vi "Set Target Node.vi"(0 "FSM.Graph In":refnum<class "FSM.Graph.lvclass">, 7 "Index":i32) -> (4 "FSM.Graph Out":refnum<class "FSM.Graph.lvclass">)   [LabVIEW 2020, in "FSM.Graph.lvclass"]
uses:
  FSM.Graph.lvclass
  FSM.Graph.lvclass/FSM.Graph.ctl
  FSM.Node/FSM.Node.lvclass/FSM.Node.ctl
  FSM.Node/Write BannerColor.vi
  FSM.Node/Read Shape.vi
  FSM.Node/FSM.Node.lvclass
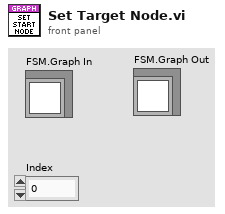
[diagram p1: front panel]
types:
  T1 = typedef "FSM.Node.lvclass/Shape.ctl" = enum16{"Default", "Start", "Action", "End"}
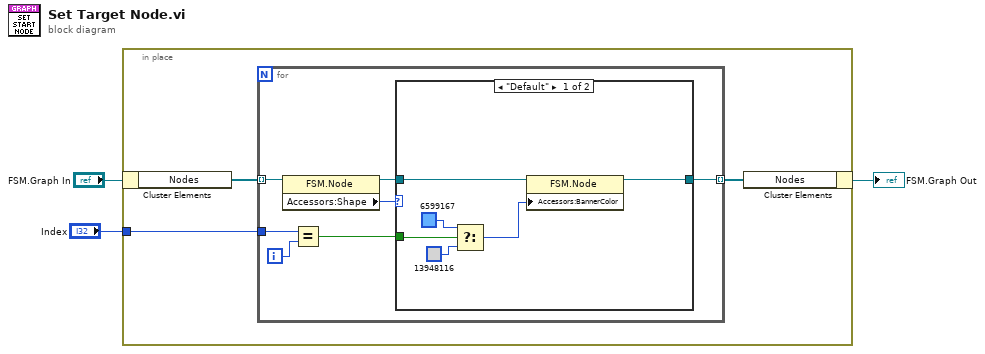
[diagram p0: block diagram]
diagram:
  n1 = in-place {
    in-place-border: "Index" -> [w5]
    n2 = in-place-cluster #1("FSM.Graph In") -> ("Nodes"=w6:refnum<class "FSM.Node.lvclass">[])
    n3 = for {
      tunnel: w6 -> [w12] mode=indexing
      tunnel: w5 -> [w13]
      tunnel: [w7] -> w4 mode=indexing
      i -> [w8]
      n4 = property class="FSM.Node"(reference=w12) -> (reference out=w10:refnum<class "FSM.Node.lvclass">, "Accessors:Shape"=w9:T1)  [unwired: 1 in, 1 out]
      n5 = Equal?(x=w13, y=w8) -> (x = y?=w11:bool)
      n6 = case shown="\"Default\"" w9 {
        tunnel: w10 -> [w19 w20]
        tunnel: [w18 w20] -> w7
        tunnel: w11 -> [w17 _]
        frame "Default" {
          n7 = Select(t=u32 6599167, s=w17, f=u32 13948116) -> (s? t:f=w15:u32)
          n8 = property class="FSM.Node"(reference=w19, "Accessors:BannerColor"=w15) -> (reference out=w18:refnum<class "FSM.Node.lvclass">)  [unwired: 1 in, 1 out]
        }
        frame "Start", Default {
        }
      }
    }
    n9 = in-place-cluster #1("Nodes"=w4) -> (→"FSM.Graph Out":refnum<class "FSM.Graph.lvclass">)
  }
